vi "Write motors.vi"(8 "error in (no error)":errorcluster, 10 "motors":refnum<class "Motor.lvclass">[](array[class]), 11 "ICS in":refnum<class "ICS.lvclass">) -> (0 "error out":errorcluster, 3 "ICS out":refnum<class "ICS.lvclass">)   [LabVIEW 2018, in "ICS.lvclass"]
uses:
  ICS.lvclass
  Motor/Motor.lvclass
  ICS.lvclass/ICS.ctl
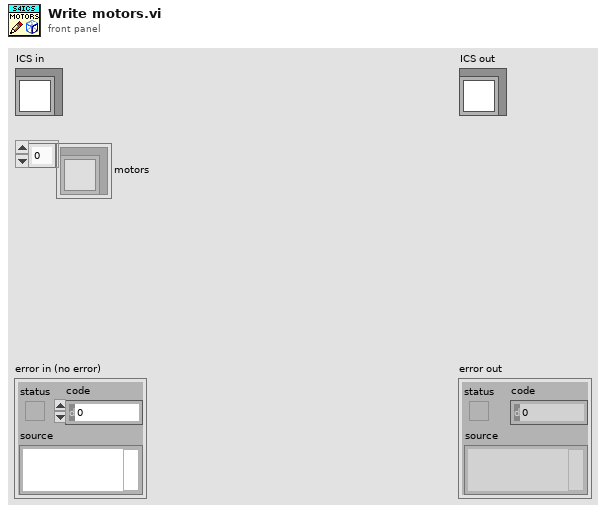
[diagram p1: front panel]
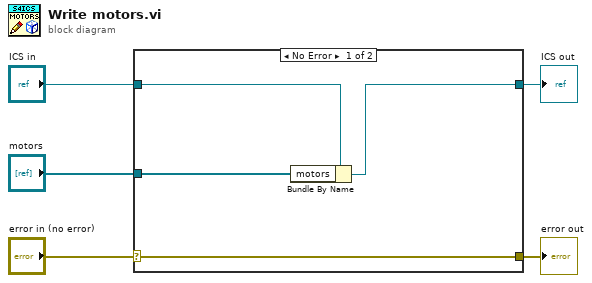
[diagram p0: block diagram]
diagram:
  n1 = case shown="No Error" "error in (no error)" {
    selector: "error in (no error)" -> [w9 w10]
    tunnel: [w9 w10] -> w4
    tunnel: [w7 w11] -> w2
    tunnel: "ICS in" -> [w8 w11]
    tunnel: "motors" -> [w6 _]
    frame No Error {
      n2 = Bundle By Name(cluster=w8, "motors"=w6) -> (w7:refnum<class "ICS.lvclass">)
    }
    frame Error {
    }
  }
  "error out" <- w4
  "ICS out" <- w2
